vi "XY Graph Get Plots to Preserve.vi"(8 "Error In":errorcluster, 10 "Default (none)":i32[](array[numeric]), 11 "XYGraph in":T1) -> (0 "Error Out":errorcluster, 1 "Preserved Plots Found?":bool, 2 "Preserved Plots":i32[](array[numeric]), 3 "XYGraph dup":T1)   [LabVIEW 2021, in "XY Graph Add-Ons.lvlib"]
uses:
  XY Graph Add-Ons.lvlib
  XY Graph Refnum.ctl
  XY Graph Property Tag List.ctl
  Variant/Variant to Data/Variant to [I32].vi
  <vilib>/UserTags/UserTags.lvlib
  Variant/Variant to Data/Variant to Data.lvlib
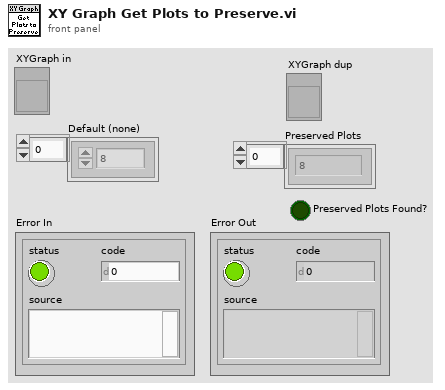
[diagram p1: front panel]
types:
  T1 = typedef "XY Graph Add-Ons.lvlib/XY Graph Refnum.ctl" = refnum<vi>
  T2 = typedef "XY Graph Add-Ons.lvlib/XY Graph Property Tag List.ctl" = enum16{"Max Legend Size", "Preserved Plots", "XScales.GridColors", "YScales.GridColors", "TipStrip String", "TipStrip Visible", "Tool Panels Visibility", "Plots Metadata"}
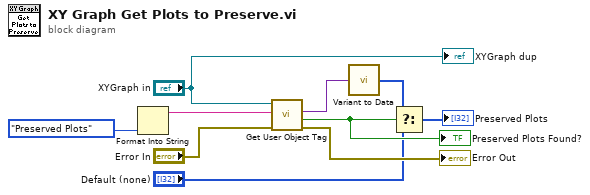
[diagram p0: block diagram]
diagram:
  n1 = Format Into String(XY_Graph_Property_Tag_List."Preserved Plots" ("XY Graph Property Tag")) -> (resulting string=w2:string)  [unwired: 3 in, 1 out]
  n2 = call <vilib>:"Get User Object Tag.vi"("error in (no error)"="Error In", "Tag Name"=w2, "Generic Refnum"="XYGraph in") -> ("error out"=→"Error Out":errorcluster, "Was Tag Found?"=w5:bool, "Value"=w8:variant)  [unwired: 5 in, 1 out]
  "Preserved Plots Found?" <- w5
  n3 = call-poly "Variant to Data.vi"("Variant"=w8) -> ("Value"=w7:i32[])  [unwired: 8 in]
  n4 = Select(t=w7, s=w5, f="Default (none)") -> (s? t:f=→"Preserved Plots":i32[])
  "XYGraph dup" <- "XYGraph in"
